vi "GoAndKickTacticVSS.vi"(5 "First call?":bool=TRUE, 8 "error in (no error)":errorcluster, 9 "Game in":refnum<class "Game.lvclass">, 10 "Robot":refnum<class "Robot.lvclass">, 11 "GoAndKickTacticVSS in":refnum<class "GoAndKickTacticVSS.lvclass">) -> (0 "error out":errorcluster, 2 "Robot out":refnum<class "Robot.lvclass">, 3 "GoAndKickTacticVSS out":refnum<class "GoAndKickTacticVSS.lvclass">, 7 "x .or. y?":bool)   [LabVIEW 2023, in "GoAndKickTacticVSS.lvclass"]
uses:
  GoAndKickTacticVSS.lvclass
  Robot_class/Robot.lvclass
  Game_class/Game.lvclass
  Robot_class/tactics.ctl
  Tactic_class/Tactic.lvclass/Tactic.ctl
  Robot_class/Robot.lvclass/Robot.ctl
  Game_class/Read BallRef.vi
  Tactic_class/Read Skillbook.vi
  Robot_class/Write tactic.vi
  Skillbook_class/Skillbook.lvclass
  KickSkillVSS_class/KickSkillVSS.lvclass
  PenaltyPosSkillVSS_class/PenaltyPosSkillVSS.lvclass
  BallDispPosSkillVSS_class/BallDispPosSkillVSS.lvclass
  BallToGoalSkillVSS_class/BallToGoalSkillVSS.lvclass
  GoToBallSkillVSS_class/GoToBallSkillVSS.lvclass
  DefBallPosSkillVSS_class/DefBallPosSkillVSS.lvclass
  HaltSkill_class/HaltSkill.lvclass
  KeeperDefPosSkillVSS_class/KeeperDefPosSkillVSS.lvclass
  GoToBallKeeperSkillVSS_class/GoToBallKeeperSkillVSS.lvclass
  RotateWallSkillVSS_class/RotateWallSkillVSS.lvclass
  Ball_class/Ball.lvclass
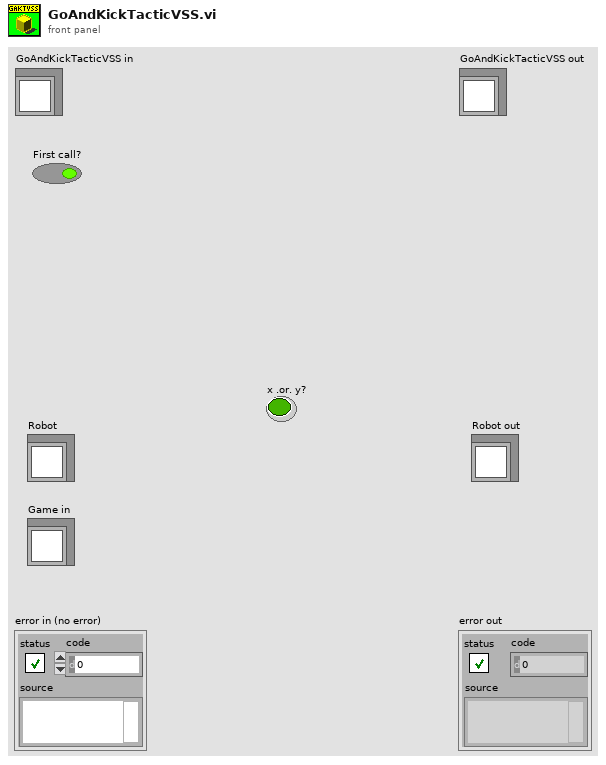
[diagram p1: front panel]
types:
  T1 = typedef "tactics.ctl" = enum16{"ReceivePassInFuturePoint", "Roller", "PrepareRollToPassRollerGoTo", "PrepareRollToPassReceiverGoTo", "WaitRoll", "PositionToRoll", "PenaltyAttacker", "PassObserver", "PenaltyDefense", "TableReceiverTactic", "Test", "DefendGoal", "Marker", "FollowAttacker", "DefendArea", "Shoot", "AttackerAimGoal", "AttackerBallOutOfField", "AttackerBlock", "AttackerStop", "Duelist", "Halt", "ZigZag", "GoTo", "Timeout", "KickToPassReceiver", "PositionToReceivePass", "DefendAreaVSS", "DefendGoalVSS", "KickVSS", "AttackVSS", "DispBallVSS", "PenaltyAttackVSS", "WaitPass"}
  T2 = cluster{"KickSkillVSS":refnum<class "KickSkillVSS.lvclass">, "PenaltyPosSkillVSS":refnum<class "PenaltyPosSkillVSS.lvclass">, "BallDispPosSkillVSS":refnum<class "BallDispPosSkillVSS.lvclass">, "BallToGoalSkillVSS":refnum<class "BallToGoalSkillVSS.lvclass">, "GoToBallSkillVSS":refnum<class "GoToBallSkillVSS.lvclass">, "DefBallPosSkillVSS":refnum<class "DefBallPosSkillVSS.lvclass">, "HaltSkill":refnum<class "HaltSkill.lvclass">, "KeeperDefPosSkillVSS":refnum<class "KeeperDefPosSkillVSS.lvclass">, "GoToBallKeeperSkillVSS":refnum<class "GoToBallKeeperSkillVSS.lvclass">, "RotateWallSkillVSS":refnum<class "RotateWallSkillVSS.lvclass">}
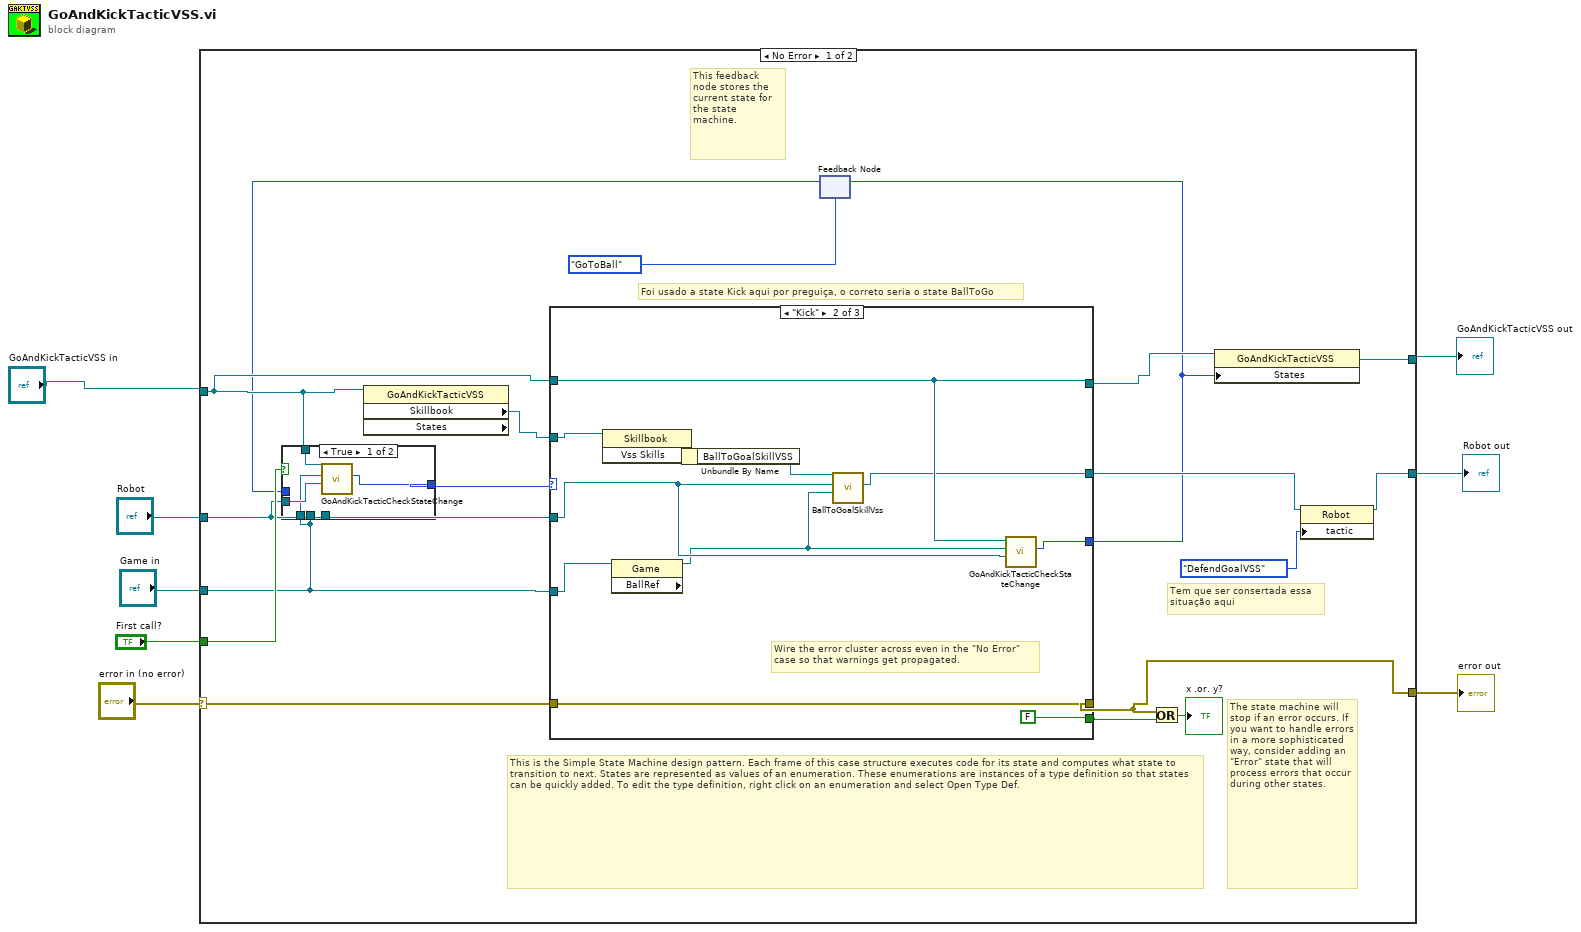
[diagram p0: block diagram]
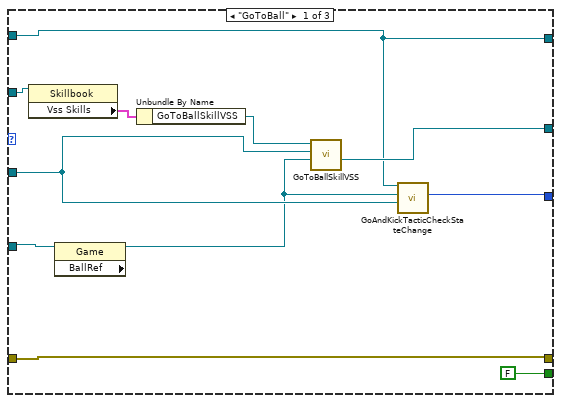
[diagram p2: hidden frame]
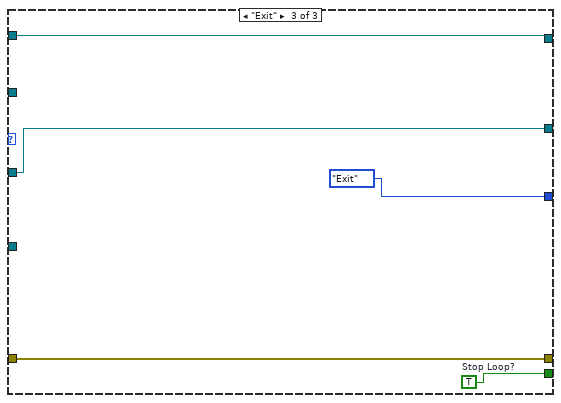
[diagram p3: hidden frame]
diagram:
  n1 = case shown="No Error" "error in (no error)" {
    selector: "error in (no error)" -> [w16 w61]
    tunnel: [w17 w61] -> w3
    tunnel: [w26 w60] -> w1
    tunnel: "GoAndKickTacticVSS in" -> [w20 w60]
    tunnel: "Robot" -> [w10 w59]
    tunnel: "Game in" -> [w9 _]
    tunnel: [w24 w59] -> w2
    tunnel: "First call?" -> [w23 _]
    frame No Error {
      # "Foi usado a state Kick aqui por preguiça, o correto seria o state BallToGo"
      # "Tem que ser consertada essa \nsituação aqui"
      # "The state machine will stop if an error occurs. If you want to handle errors in a more sophisticated way, consider adding an \"Error\" state that will process errors that occur during other states."
      # "This feedback node stores the current state for the state machine."
      # "This is the Simple State Machine design pattern. Each frame of this case structure executes code for its state and computes what state to transition to next. States are represented as values of an enumeration. These enumerations are instances of a type definition so that states can be quickly added. To edit the type definition, right click on an enumeration and select Open Type Def."
      n2 = property class="GoAndKickTacticVSS" props=["Skillbook", "States"](reference=w20) -> ("Skillbook"=w15:refnum<class "Skillbook.lvclass">)  [unwired: 1 in, 3 out]
      n3 = feedback #1(enum16{"GoToBall", "Kick", "Exit"}."GoToBall" ("States")) -> (w12:enum16{"GoToBall", "Kick", "Exit"})
      n4 = case shown="True" w23 {
        tunnel: w20 -> [w57 _]
        tunnel: w10 -> [_ _]
        tunnel: w9 -> [_ _]
        tunnel: [w56 w58] -> w13
        tunnel: w12 -> [_ w58]
        tunnel: w10 -> [w55 _]
        tunnel: w9 -> [w54 _]
        frame True {
          n5 = call "GoAndKickTacticCheckStateChange.vi"("Robot In"=w55, "Game in"=w54, "GoAndKickTacticVSS in"=w57) -> ("States"=w56:enum16{"GoToBall", "Kick", "Exit"})  [unwired: 6 in, 2 out]
        }
        frame False {
        }
      }
      n6 = case shown="\"Kick\"" w13 {
        tunnel: w9 -> [w35 w46 _]
        tunnel: w10 -> [w28 w40 w51]
        tunnel: [w34 w38 w51] -> w21
        tunnel: w20 -> [w33 w45 w50]
        tunnel: [w33 w45 w50] -> w19
        tunnel: [w29 w44 enum16{"GoToBall", "Kick", "Exit"}."Exit" ("States")] -> w11
        tunnel: [FALSE ("Stop Loop?") FALSE ("Stop Loop?") w52] -> w18
        tunnel: [w32 w43 w53] -> w17
        tunnel: w16 -> [w32 w43 w53]
        tunnel: w15 -> [w31 w47 _]
        frame "GoToBall" {
          n7 = property class="Skillbook"(reference=w31) -> ("Vss Skills"=w37:T2)  [unwired: 1 in, 2 out]
          n8 = property class="Game" props=["BallRef"](reference=w35) -> (reference out=w27:refnum<class "Game.lvclass">)  [unwired: 1 in, 2 out]
          n9 = Unbundle By Name(w37) -> ("GoToBallSkillVSS"=w36:refnum<class "GoToBallSkillVSS.lvclass">)
          n10 = call "GoToBallSkillVSS.vi"("Game"=w27, "Robot in"=w28, "GoToBallSkillVSS in"=w36) -> ("Robot out"=w34:refnum<class "Robot.lvclass">)  [unwired: 6 in, 2 out]
          n11 = call "GoAndKickTacticCheckStateChange.vi"("Robot In"=w28, "Game in"=w27, "GoAndKickTacticVSS in"=w33) -> ("States"=w29:enum16{"GoToBall", "Kick", "Exit"})  [unwired: 6 in, 2 out]
        }
        frame "Kick" {
          # "Wire the error cluster across even in the \"No Error\"\ncase so that warnings get propagated."
          n12 = property class="Skillbook"(reference=w47) -> ("Vss Skills"=w48:T2)  [unwired: 1 in, 2 out]
          n13 = property class="Game" props=["BallRef"](reference=w46) -> (reference out=w39:refnum<class "Game.lvclass">)  [unwired: 1 in, 2 out]
          n14 = Unbundle By Name(w48) -> ("BallToGoalSkillVSS"=w41:refnum<class "BallToGoalSkillVSS.lvclass">)
          n15 = call "BallToGoalSkillVss.vi"("Game"=w39, "Robot in"=w40, "BallToGoalSkillVSS in"=w41) -> ("Robot out"=w38:refnum<class "Robot.lvclass">)  [unwired: 6 in, 2 out]
          n16 = call "GoAndKickTacticCheckStateChange.vi"("Robot In"=w40, "Game in"=w39, "GoAndKickTacticVSS in"=w45) -> ("States"=w44:enum16{"GoToBall", "Kick", "Exit"})  [unwired: 6 in, 2 out]
        }
        frame "Exit" {
          w52 = TRUE  # Stop Loop?
        }
      }
      n17 = feedback-in #1(w11) -> ()
      n18 = Or(x=w17, y=w18) -> (x .or. y?=→"x .or. y?":bool)
      n19 = property class="GoAndKickTacticVSS"(reference=w19, "States"=w11) -> (reference out=w26:refnum<class "GoAndKickTacticVSS.lvclass">)  [unwired: 1 in, 1 out]
      n20 = property class="Robot"(reference=w21, "tactic"=tactics."DefendGoalVSS") -> (reference out=w24:refnum<class "Robot.lvclass">)  [unwired: 1 in, 1 out]
    }
    frame Error {
    }
  }
  "error out" <- w3
  "Robot out" <- w2
  "GoAndKickTacticVSS out" <- w1
